vi "3D Chop One Bin.vi"(4 "tolerance":dbl=1e-16, 6 "VI ref":cluster{"f(x)":refnum<vi>, "data":variant}, 7 "Formula":T1, 8 "error in (no error)":errorcluster, 9 "Formula/VI ref":bool, 10 "chop x?":bool, 11 "Bins In":T3={"bin x"={"lower limit"=0.0, "upper limit"=1.0}, "bin y"={"lower limit"=0.0, "upper limit"=1.0}, "bin z"={"lower limit"=0.0, "upper limit"=1.0}}) -> (0 "error out":errorcluster, 2 "Chop x Out":bool[](array[boolean]), 3 "Bins Out":T2(array[cluster]))   [LabVIEW 2017, in "NI_AALPro.lvlib"]
uses:
  NI_AALPro.lvlib
  A x Vector.vi
  Real Dot Product.vi
  NI_AALBase.lvlib
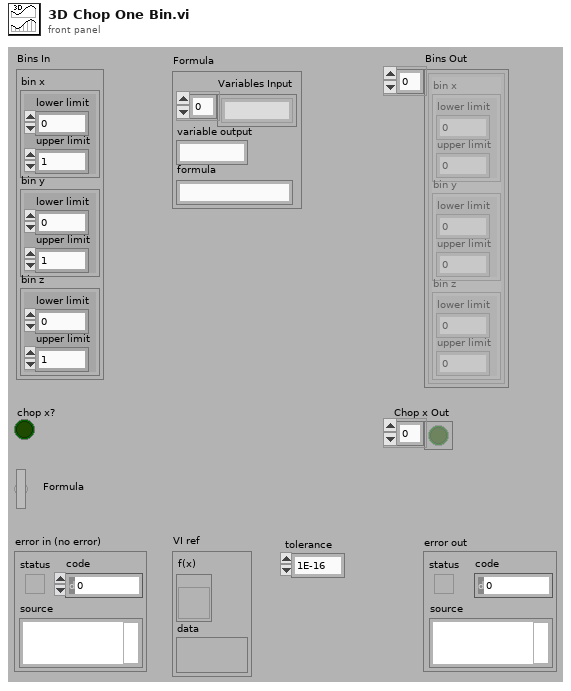
[diagram p1: front panel]
types:
  T1 = cluster{"Variables Input":string[], "variable output":string, "formula":string}
  T2 = cluster{"bin x":cluster{"lower limit":dbl, "upper limit":dbl}, "bin y":cluster{"lower limit":dbl, "upper limit":dbl}, "bin z":cluster{"lower limit":dbl, "upper limit":dbl}}[]
  T3 = cluster{"bin x":cluster{"lower limit":dbl, "upper limit":dbl}, "bin y":cluster{"lower limit":dbl, "upper limit":dbl}, "bin z":cluster{"lower limit":dbl, "upper limit":dbl}}
  T4 = cluster{"bin_x":cluster{"lower limit":dbl, "upper limit":dbl}, "bin_y":cluster{"lower limit":dbl, "upper limit":dbl}, "bin_z":cluster{"lower limit":dbl, "upper limit":dbl}}[]
  T5 = cluster{cluster{dbl, dbl}, cluster{dbl, dbl}, cluster{dbl, dbl}}
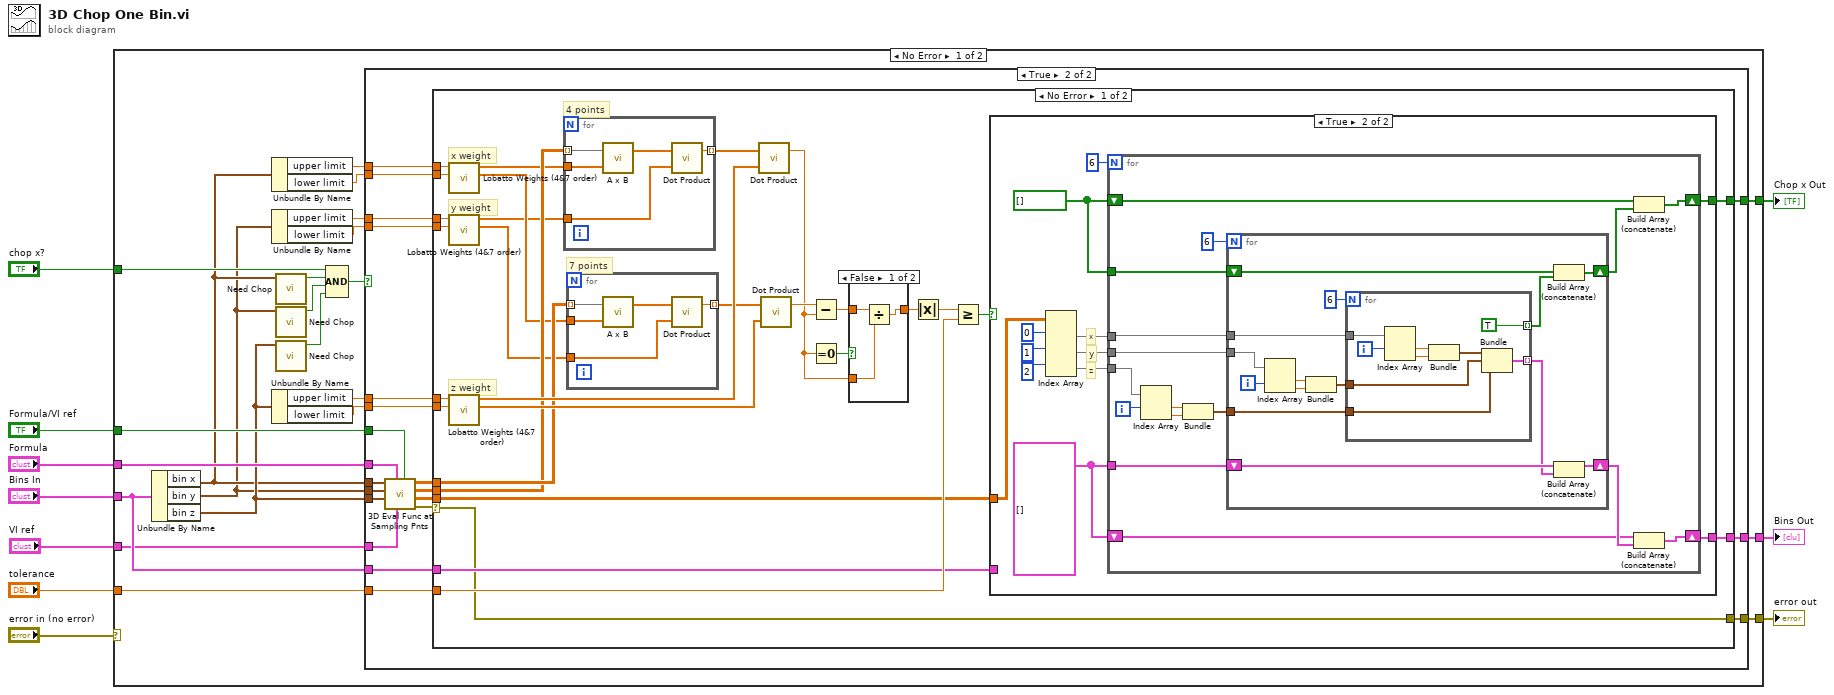
[diagram p0: block diagram]
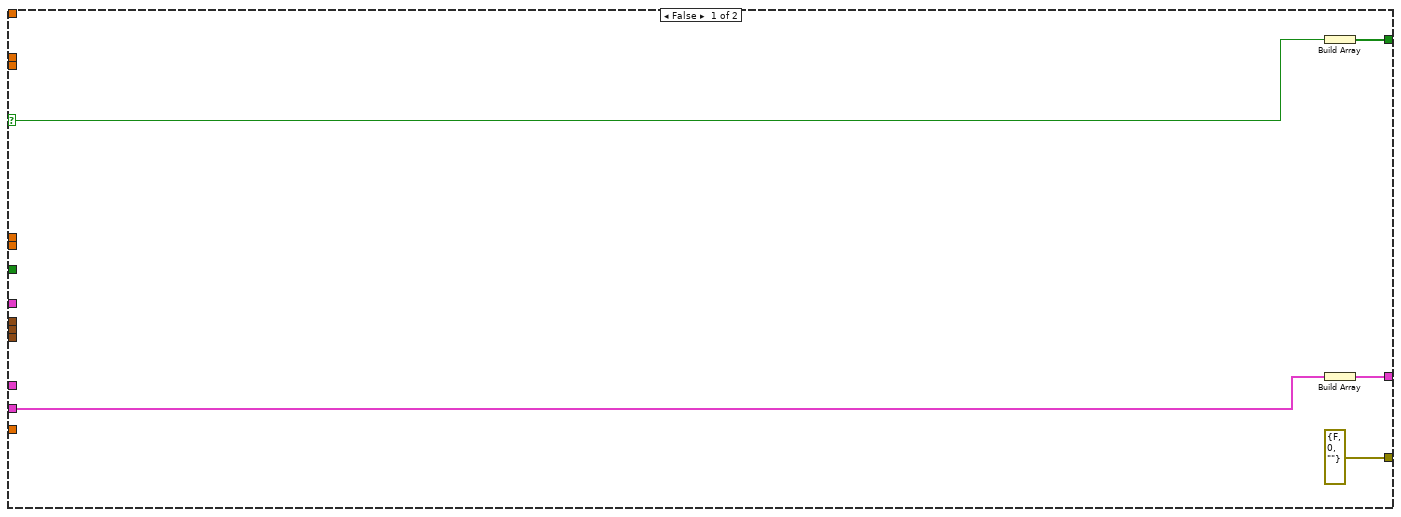
[diagram p2: hidden frame]
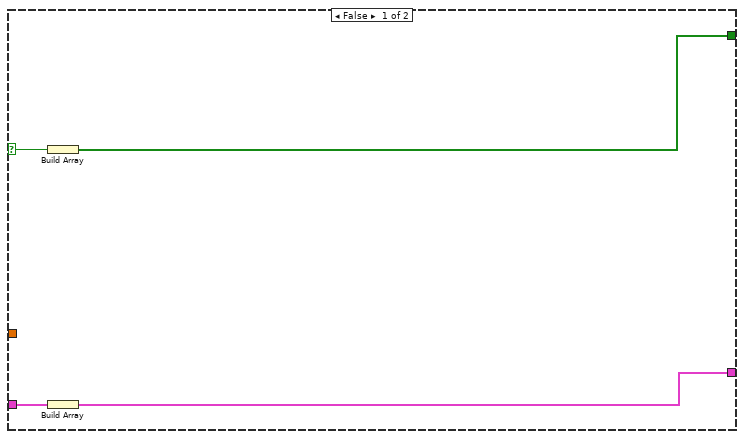
[diagram p4: hidden frame]
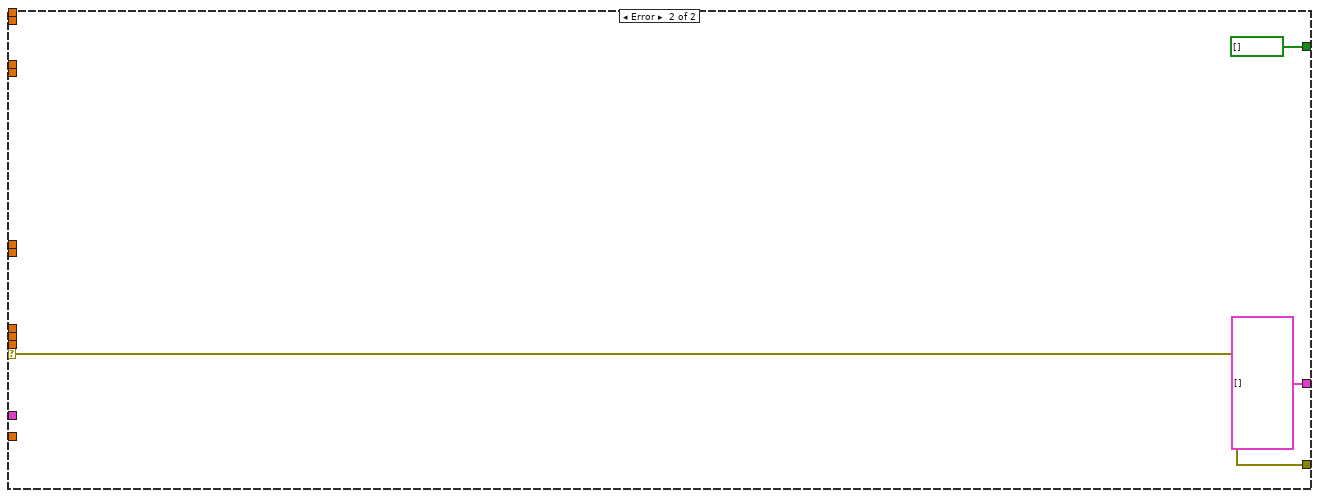
[diagram p5: hidden frame]
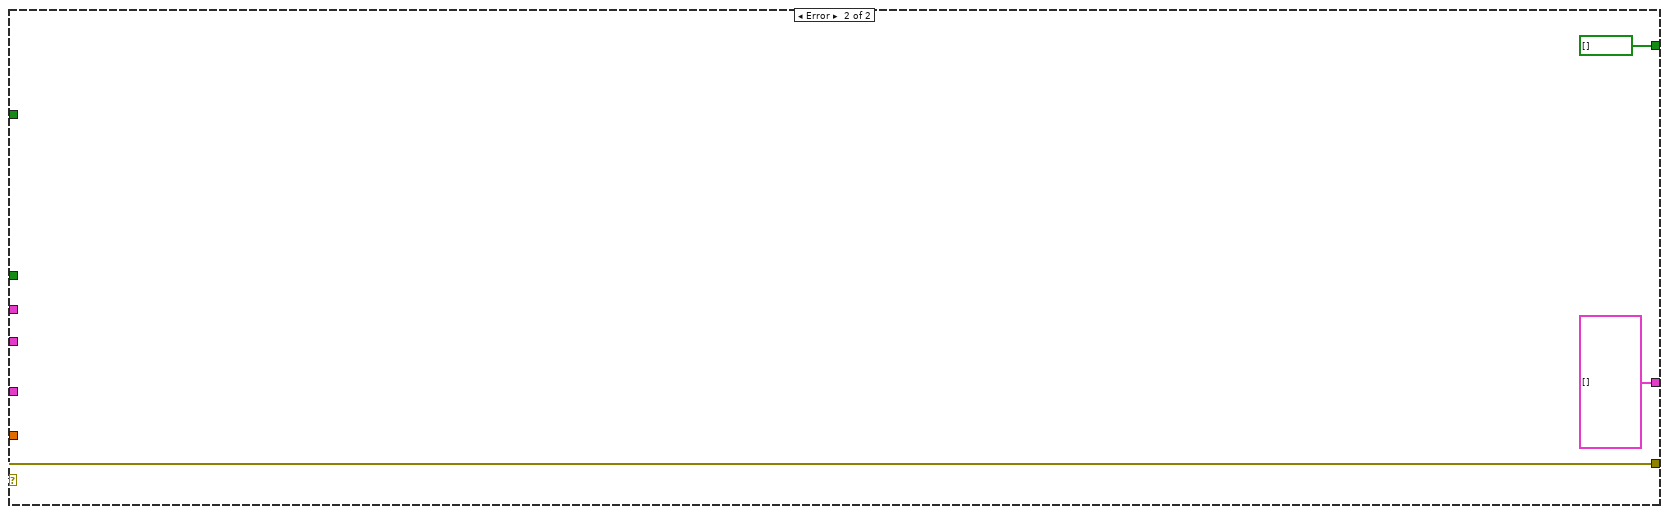
[diagram p6: hidden frame]
diagram:
  n1 = case shown="No Error" "error in (no error)" {
    selector: "error in (no error)" -> [_ w162]
    tunnel: "Bins In" -> [w28 _]
    tunnel: "tolerance" -> [w27 _]
    tunnel: [w26 bool[] [] ("Chop x Out")] -> w8
    tunnel: [w25 T4 [] ("Bins Out")] -> w7
    tunnel: [w24 w162] -> w6
    tunnel: "VI ref" -> [w23 _]
    tunnel: "Formula/VI ref" -> [w22 _]
    tunnel: "Formula" -> [w21 _]
    tunnel: "chop x?" -> [w20 _]
    frame No Error {
      n2 = Unbundle By Name(w28) -> ("bin x"=w18:cluster{"lower limit":dbl, "upper limit":dbl}, "bin y"=w17:cluster{"lower limit":dbl, "upper limit":dbl}, "bin z"=w19:cluster{"lower limit":dbl, "upper limit":dbl})
      n3 = Unbundle By Name(w18) -> ("upper limit"=w15:dbl, "lower limit"=w32:dbl)
      n4 = Unbundle By Name(w17) -> ("upper limit"=w30:dbl, "lower limit"=w16:dbl)
      n5 = Unbundle By Name(w19) -> ("upper limit"=w29:dbl, "lower limit"=w14:dbl)
      n6 = call "Need Chop.vi"("bin"=w18) -> ("chop?"=w13:bool)  [unwired: 10 out]
      n7 = call "Need Chop.vi"("bin"=w17) -> ("chop?"=w12:bool)  [unwired: 10 out]
      n8 = call "Need Chop.vi"("bin"=w19) -> ("chop?"=w11:bool)  [unwired: 10 out]
      n9 = Compound Arithmetic op=AND(w20, w13, w12, w11) -> (w31:bool)
      n10 = case shown="True" w31 {
        selector: w31 -> [w37 _]
        tunnel: [w35 w56] -> w25
        tunnel: [w36 w55] -> w26
        tunnel: w32 -> [_ w53]
        tunnel: w15 -> [_ w52]
        tunnel: w27 -> [_ w54]
        tunnel: [errorcluster {"status"=FALSE, "code"=0, "source"=""} ("error out") w38] -> w24
        tunnel: w18 -> [_ w51]
        tunnel: w17 -> [_ w50]
        tunnel: w16 -> [_ w49]
        tunnel: w30 -> [_ w48]
        tunnel: w28 -> [w33 w47]
        tunnel: w19 -> [_ w46]
        tunnel: w29 -> [_ w45]
        tunnel: w14 -> [_ w44]
        tunnel: w23 -> [_ w42]
        tunnel: w22 -> [_ w41]
        tunnel: w21 -> [_ w40]
        frame False {
          n11 = Build Array(w37) -> (w36:bool[])
          n12 = Build Array(w33) -> (w35:T2)
        }
        frame True {
          n13 = call "3D Eval Func at Sampling Pnts.vi"("Formula/VI ref"=w41, "VI ref"=w42, "Formula"=w40, "z limit"=w46, "y limit"=w50, "x limit"=w51) -> ("error out"=w39:errorcluster, "Sampling points (7-order)"=w43:dbl[][], "Function Evaluations (4 pts)"=w57:dbl[][][], "Function Evaluations (7 pts)"=w58:dbl[][][])  [unwired: 1 in, 1 out]
          n14 = case shown="No Error" w39 {
            selector: w39 -> [w59 w157]
            tunnel: w58 -> [w85 _]
            tunnel: w57 -> [w84 _]
            tunnel: [w82 T4 [] ("Bins Out")] -> w56
            tunnel: [w81 bool[] [] ("Chop x Out")] -> w55
            tunnel: w54 -> [w80 _]
            tunnel: w53 -> [w76 _]
            tunnel: w52 -> [w75 _]
            tunnel: w49 -> [w73 _]
            tunnel: w48 -> [w72 _]
            tunnel: w47 -> [w68 _]
            tunnel: w45 -> [w67 _]
            tunnel: w44 -> [w66 _]
            tunnel: w43 -> [w64 _]
            tunnel: [w59 w157] -> w38
            frame No Error {
              # "7 points"
              # "4 points"
              # "z weight"
              # "y weight"
              # "x weight"
              n15 = call "Lobatto Weights (4&7 order).vi"("lower limit"=w76, "upper limit"=w75) -> ("Weights (7-Order)"=w74:dbl[], "Weights (4-Order)"=w71:dbl[])  [unwired: 8 out]
              n16 = call "Lobatto Weights (4&7 order).vi"("lower limit"=w73, "upper limit"=w72) -> ("Weights (7-Order)"=w65:dbl[], "Weights (4-Order)"=w70:dbl[])  [unwired: 8 out]
              n17 = call "Lobatto Weights (4&7 order).vi"("lower limit"=w66, "upper limit"=w67) -> ("Weights (7-Order)"=w87:dbl[], "Weights (4-Order)"=w86:dbl[])  [unwired: 8 out]
              n18 = for {
                tunnel: w84 -> [w90] mode=indexing
                tunnel: w71 -> [w89]
                tunnel: w70 -> [w92]
                tunnel: [w91] -> w62 mode=indexing
                n19 = call-poly "A x B.vi"("Vector"=w89, "A"=w90) -> ("A x Vector"=w88:dbl[])  [unwired: 1 out]
                n20 = call-poly "Dot Product.vi"("Y Vector"=w92, "X Vector"=w88) -> ("X * Y"=w91:dbl)  [unwired: 1 out]
              }
              n21 = for {
                tunnel: w85 -> [w95] mode=indexing
                tunnel: w74 -> [w94]
                tunnel: w65 -> [w96]
                tunnel: [w97] -> w60 mode=indexing
                n22 = call-poly "A x B.vi"("Vector"=w94, "A"=w95) -> ("A x Vector"=w93:dbl[])  [unwired: 1 out]
                n23 = call-poly "Dot Product.vi"("Y Vector"=w96, "X Vector"=w93) -> ("X * Y"=w97:dbl)  [unwired: 1 out]
              }
              n24 = call-poly "Dot Product.vi"("Y Vector"=w86, "X Vector"=w62) -> ("X * Y"=w61:dbl)  [unwired: 1 out]
              n25 = call-poly "Dot Product.vi"("Y Vector"=w87, "X Vector"=w60) -> ("X * Y"=w63:dbl)  [unwired: 1 out]
              n26 = Subtract(x=w63, y=w61) -> (x-y=w78:dbl)
              n27 = Equal To 0?(x=w61) -> (x = 0?=w79:bool)
              n28 = case shown="False" w79 {
                tunnel: w78 -> [w100 w101]
                tunnel: w61 -> [w99 _]
                tunnel: [w98 w101] -> w77
                frame False {
                  n29 = Divide(x=w100, y=w99) -> (x/y=w98:dbl)
                }
                frame True {
                }
              }
              n30 = Absolute Value(x=w77) -> (abs(x)=w69:dbl)
              n31 = Greater Or Equal?(x=w69, y=w80) -> (x >= y?=w83:bool)
              n32 = case shown="True" w83 {
                selector: w83 -> [w103 _]
                tunnel: w64 -> [_ w117]
                tunnel: [w104 w112] -> w82
                tunnel: w68 -> [w105 _]
                tunnel: [w102 w108] -> w81
                frame False {
                  n33 = Build Array(w103) -> (w102:bool[])
                  n34 = Build Array(w105) -> (w104:T2)
                }
                frame True {
                  w106 = bool[] [] ("Chop x Out")
                  w107 = T4 [] ("Bins Out")
                  # "z"
                  # "y"
                  # "x"
                  n35 = Index Array(array=w117, index (row) #1=0 ("index (row)"), index (row) #2=1 ("index (row)"), index (row) #3=2 ("index (row)")) -> (element #1=w116:dbl[], element #2=w113:dbl[], element #3=w110:dbl[])  [unwired: 3 in]
                  n36 = for {
                    N: 6 -> [_]
                    tunnel: w116 -> [w133]
                    tunnel: w113 -> [w132]
                    tunnel: w110 -> [w129]
                    shift-right: [w126] -> w108
                    shift-left: w106 -> [w127]
                    shift-right: [w123] -> w112
                    shift-left: w107 -> [w124]
                    tunnel: w107 -> [w122]
                    tunnel: w106 -> [w121]
                    i -> [w130]
                    n37 = Index Array(array=w129, index #1=w130) -> (element #1=w120:dbl, element #2=w119:dbl)  [unwired: 1 in]
                    n38 = Bundle(w120, w119) -> (w118:cluster{dbl, dbl})  [unwired: 1 out]
                    n39 = for {
                      N: 6 -> [_]
                      tunnel: w133 -> [w147]
                      tunnel: w132 -> [w145]
                      shift-right: [w141] -> w128
                      shift-left: w121 -> [w144]
                      shift-right: [w138] -> w125
                      shift-left: w122 -> [w143]
                      tunnel: w118 -> [w137]
                      i -> [w146]
                      n40 = Index Array(array=w145, index #1=w146) -> (element #1=w136:dbl, element #2=w135:dbl)  [unwired: 1 in]
                      n41 = Bundle(w136, w135) -> (w134:cluster{dbl, dbl})  [unwired: 1 out]
                      n42 = for {
                        N: 6 -> [_]
                        tunnel: w147 -> [w156]
                        tunnel: [TRUE] -> w140 mode=indexing
                        tunnel: [w150] -> w142 mode=indexing
                        tunnel: w137 -> [w149]
                        tunnel: w134 -> [w148]
                        i -> [w155]
                        n43 = Index Array(array=w156, index #1=w155) -> (element #1=w153:dbl, element #2=w154:dbl)  [unwired: 1 in]
                        n44 = Bundle(w153, w154) -> (w151:cluster{dbl, dbl})  [unwired: 1 out]
                        n45 = Bundle(w151, w148, w149) -> (w150:T5)  [unwired: 1 out]
                      }
                      n46 = Build Array (concatenate)(w144, w140) -> (w141:bool[])
                      n47 = Build Array (concatenate)(w143, w142) -> (w138:T4)
                    }
                    n48 = Build Array (concatenate)(w127, w128) -> (w126:bool[])
                    n49 = Build Array (concatenate)(w124, w125) -> (w123:T4)
                  }
                }
              }
            }
            frame Error {
            }
          }
        }
      }
    }
    frame Error {
    }
  }
  "Chop x Out" <- w8
  "error out" <- w6
  "Bins Out" <- w7
